vi "readSettingsFile.vi"(8 "error in (no error)":errorcluster, 11 "Controller.LV in":refnum<class "Controller.LV.lvclass">) -> (0 "error out":errorcluster, 3 "Controller.LV out":refnum<class "Controller.LV.lvclass">)   [LabVIEW 2019, in "Controller.LV.lvclass"]
uses:
  Controller.LV.lvclass
  drivers/Class/Controller/Controller.lvclass
panel:
  out "Command":string
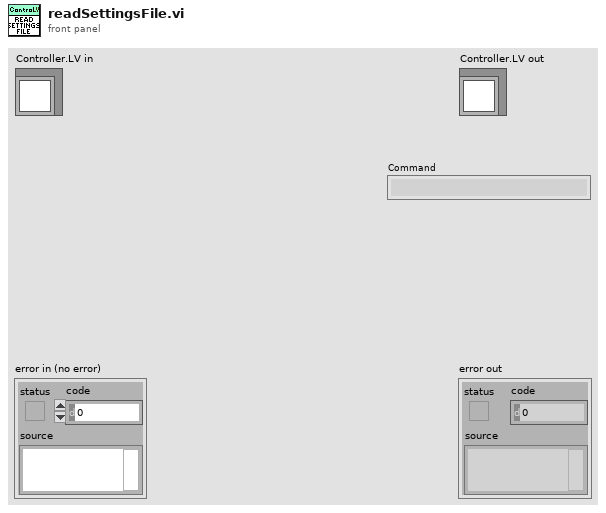
[diagram p1: front panel]
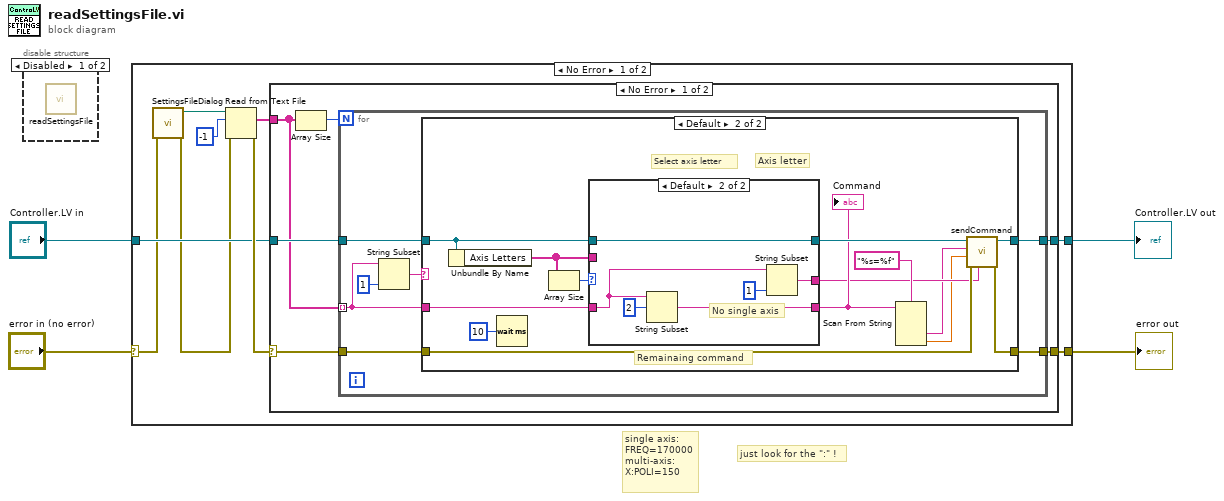
[diagram p0: block diagram]
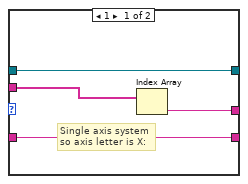
[diagram p4: hidden frame]
diagram:
  # "just look for the \":\" !"
  # "single axis:\nFREQ=170000\nmulti-axis:\nX:POLI=150"
  n1 = disable-structure shown="Disabled" {
    frame Disabled {
      n2 = call-parent "readSettingsFile.vi"() -> ()  [unwired: 10 in, 2 out]
    }
    frame Enabled {
    }
  }
  n3 = case shown="No Error" "error in (no error)" {
    selector: "error in (no error)" -> [w6 w56]
    tunnel: [w12 w56] -> w3
    tunnel: [w9 w55] -> w1
    tunnel: "Controller.LV in" -> [w10 w55]
    frame No Error {
      n4 = call "SettingsFileDialog.vi"("error in (no error)"=w6) -> ("error out"=w5:errorcluster, "selected path"=w8:path)  [unwired: 9 in]
      n5 = Read from Text File(file (use dialog)=w8, count=-1, error in=w5) -> (text=w7:string[], error out=w11:errorcluster)  [unwired: 1 in, 2 out]
      n6 = case shown="No Error" w11 {
        selector: w11 -> [w17 w54]
        tunnel: [w18 w54] -> w12
        tunnel: w10 -> [w16 w53]
        tunnel: [w15 w53] -> w9
        tunnel: w7 -> [w14 _]
        frame No Error {
          n7 = Array Size(array=w14) -> (size(s)=w19:i32)
          n8 = for {
            N: w19 -> [_]
            tunnel: w14 -> [w21] mode=indexing
            tunnel: w16 -> [w24]
            tunnel: [w23] -> w15
            tunnel: w17 -> [w26]
            tunnel: [w25] -> w18
            n9 = String Subset(string=w21, length (rest)=1 ("length (rest)")) -> (substring=w22:string)  [unwired: 1 in]
            n10 = case shown="Default" w22 {
              tunnel: w26 -> [w28 w41]
              tunnel: [w28 w40] -> w25
              tunnel: w24 -> [w27 w36]
              tunnel: [w27 w42] -> w23
              tunnel: w21 -> [_ w38]
              frame "", "%" {
                # "ignore empty lines and comments"
              }
              frame Default {
                # "Remainaing command"
                # "Axis letter"
                # "Select axis letter"
                n11 = Unbundle By Name(w36) -> ("Axis Letters"=w34:string[])
                n12 = Wait (ms)(milliseconds to wait=u32 10) -> ()  [unwired: 1 out]
                n13 = Array Size(array=w34) -> (size(s)=w35:i32)
                n14 = case shown="Default" w35 {
                  tunnel: w38 -> [w46 w48]
                  tunnel: [w46 w49] -> w33
                  tunnel: [w43 w51] -> w31
                  tunnel: w36 -> [w45 w47]
                  tunnel: [w45 w47] -> w37
                  tunnel: w34 -> [w44 _]
                  frame 1 {
                    # "Single axis system \nso axis letter is X:"
                    n15 = Index Array(array=w44) -> (element=w43:string)  [unwired: 1 in]
                  }
                  frame Default {
                    # "No single axis"
                    n16 = String Subset(string=w48, offset (0)=2) -> (substring=w49:string)  [unwired: 1 in]
                    n17 = String Subset(string=w48, length (rest)=1) -> (substring=w51:string)  [unwired: 1 in]
                  }
                }
                "Command" <- w33
                n18 = Scan From String(format string="%s=%f", input string=w33) -> (output 1=w30:string, output 2=w29:dbl)  [unwired: 4 in, 3 out]
                n19 = call-dynamic "sendCommand.vi"("Axis Letter"=w31, "error in (no error)"=w41, "Value"=w29, "Command"=w30, "Controller in"=w37) -> ("error out"=w40:errorcluster, "Controller out"=w42:refnum<class "Controller.LV.lvclass">)  [unwired: 5 in]
              }
            }
          }
        }
        frame Error {
        }
      }
    }
    frame Error {
    }
  }
  "error out" <- w3
  "Controller.LV out" <- w1
